vi "MesuresValiseCustomNeMarchePas.vi"() -> ()   [LabVIEW 2017]
uses:
  Globals/VarGlobUIStopLoops.vi
  <resource>/objmgr/daqmx.rc
  DefDeType/WhichPath.ctl
  <vilib>/DAQmx/write.llb/DAQmx Write (Digital Bool 1Line 1Point).vi
  <vilib>/DAQmx/create/channels.llb/DAQmx Create Channel (DO-Digital Output).vi
  DefDeType/ClusterRefCtrl.ctl
  <vilib>/DAQmx/read.llb/DAQmx Read (Analog 1D Wfm NChan NSamp).vi
panel:
  in  "Reprocess":bool
  in  "Next Test":u32
  out "AcqTime(s)":u16(slide) scale=0.0..1000.0
  out "Recording":bool
  in  "EnregistrerPtEtal":bool
  out "Projet":string
  in  "Essais réalisés":i32(listbox)
  out "Reload Config":bool
  out "Graph2":dbl[][](graph)
  in  "ChangerConfig":bool
  out "iterationMonitoringLoop":i32
  out "iterationEventLoop":i32
  in  "Stop Enreg.":bool
  in  "Enregistrer":bool
  out "Graph1":waveform(dbl)[](graph)
  in  "Quitter":bool
  # "Commandes"
  # "Graph 1"
  # "Essais Réalisés"
  # "Graph 2"
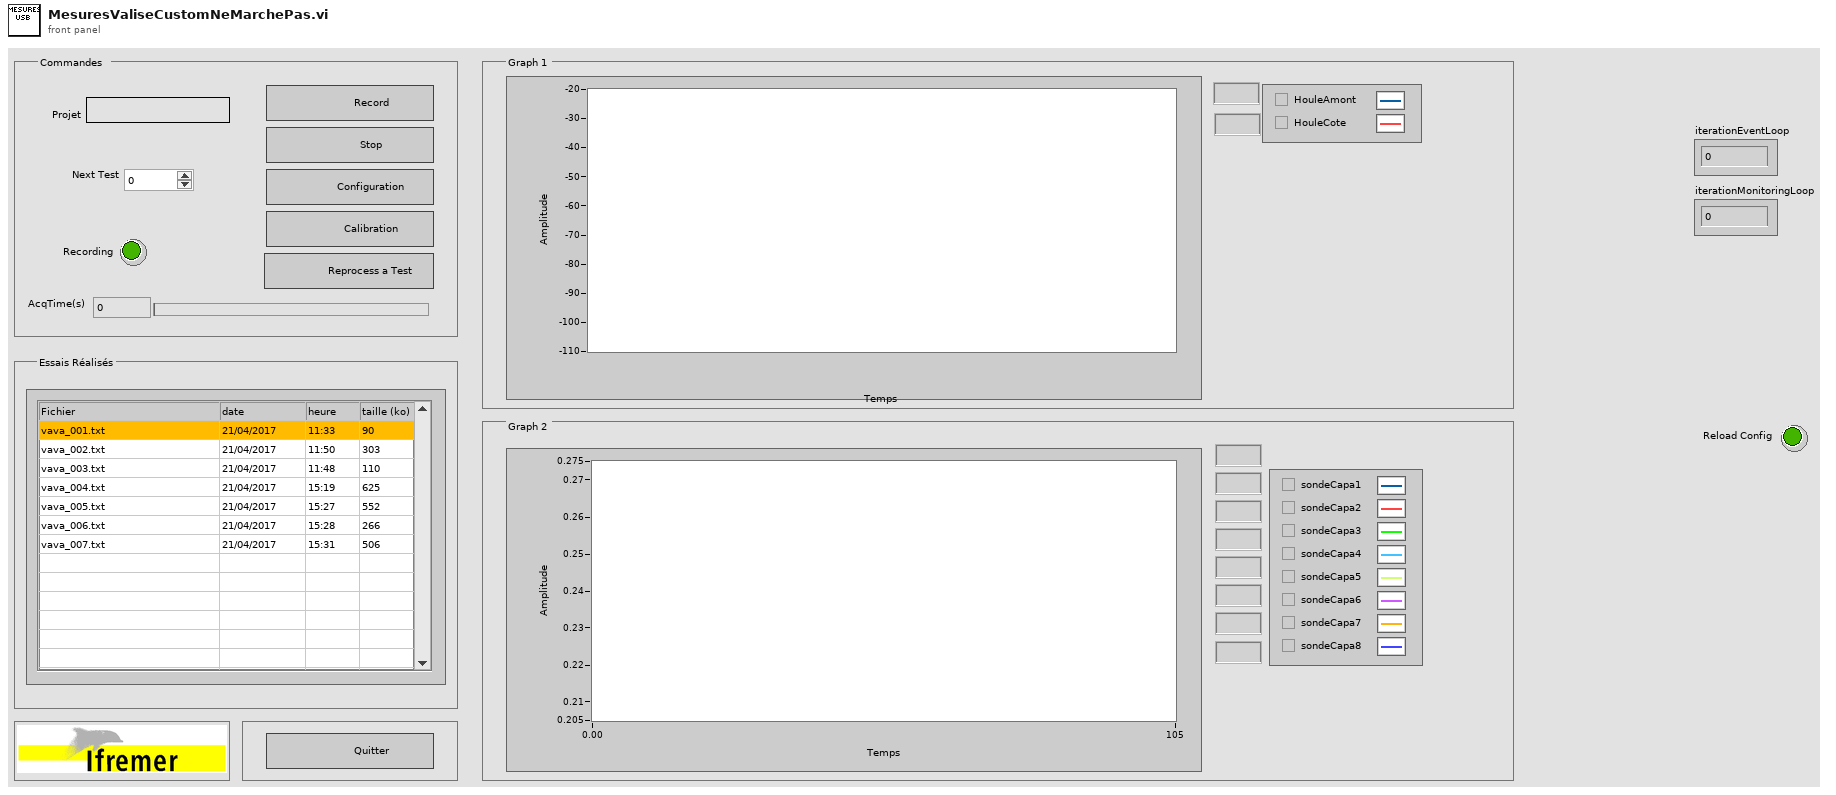
[diagram p1: front panel]
types:
  T1 = enum8{"Enabled", "Disabled", "Disabled and Grayed Out"}
  T2 = typedef "ClusterRefCtrl.ctl" = cluster{"Essais réalisés":refnum<vi>, "EnregistrerPtEtal":refnum<vi>, "ChangerConfig":refnum<vi>, "Enregistrer":refnum<vi>, "Reprocess":refnum<vi>}
  T3 = cluster{"AcqTime(s)":refnum<vi>, "Graph2":refnum<vi>, "Graph1":refnum<vi>}
  T4 = typedef "ConfigTotale.ctl" = cluster{"VoltageChannels":T5, "WheastoneBridgeChannels":T6, "Configuration":T7}
  T5 = typedef "VoltageChannels.ctl" = cluster{"ChannelNames":string[], "Sensitivity(Unit/V)":dbl[], "AutoZero":bool[], "ChannelUnits":string[], "Offsets(Units)":dbl[], "Graph Num":u8[]}
  T6 = typedef "WBridgeChannels.ctl" = cluster{"ChannelNames":string[], "Sensitivity(Unit/V)":dbl[], "AutoZero":bool[], "ChannelUnits":string[], "Offsets(Units)":dbl[], "Graph Num":u8[]}
  T7 = typedef "Configuration.ctl" = cluster{"AcqSamplingRate(Hz)":u32, "AcqTime(s)":u32, "Trigger":bool, "NbVoltageChannels":u32, "NbWBridgeChannels":u32, "Qualisys":bool, "Hexapode":bool, "FinalSamplingRate(Hz)":u32, "QualisysDataType":enum16{"6DOF", "3DTracking", "6DOF + 3D"}, "Nortek":bool, "HBM":bool}
  T8 = cluster{"Graph2Index":i32[], "Graph1Index":i32[]}
  T9 = typedef "WhichPath.ctl" = enum16{"DossierProjet", "Config", "Meas", "MeasPCI", "MeasCRIO1", "MeasCRIO2", "MeasQualisys", "MeasHBM", "MeasTDMS", "Fig", "Res"}
  T10 = typedef "MergeFileConfig.ctl" = cluster{"Test Num : ":u32, "Project :":string, "Qualisys file":path, "Hexapod file":path, "ADV Nortek file":path, "QualisysDataType":enum16{"6DOF", "3DTracking", "6DOF + 3D"}, "Qualisys":bool, "Hexapode":bool, "ADV Nortek":bool}
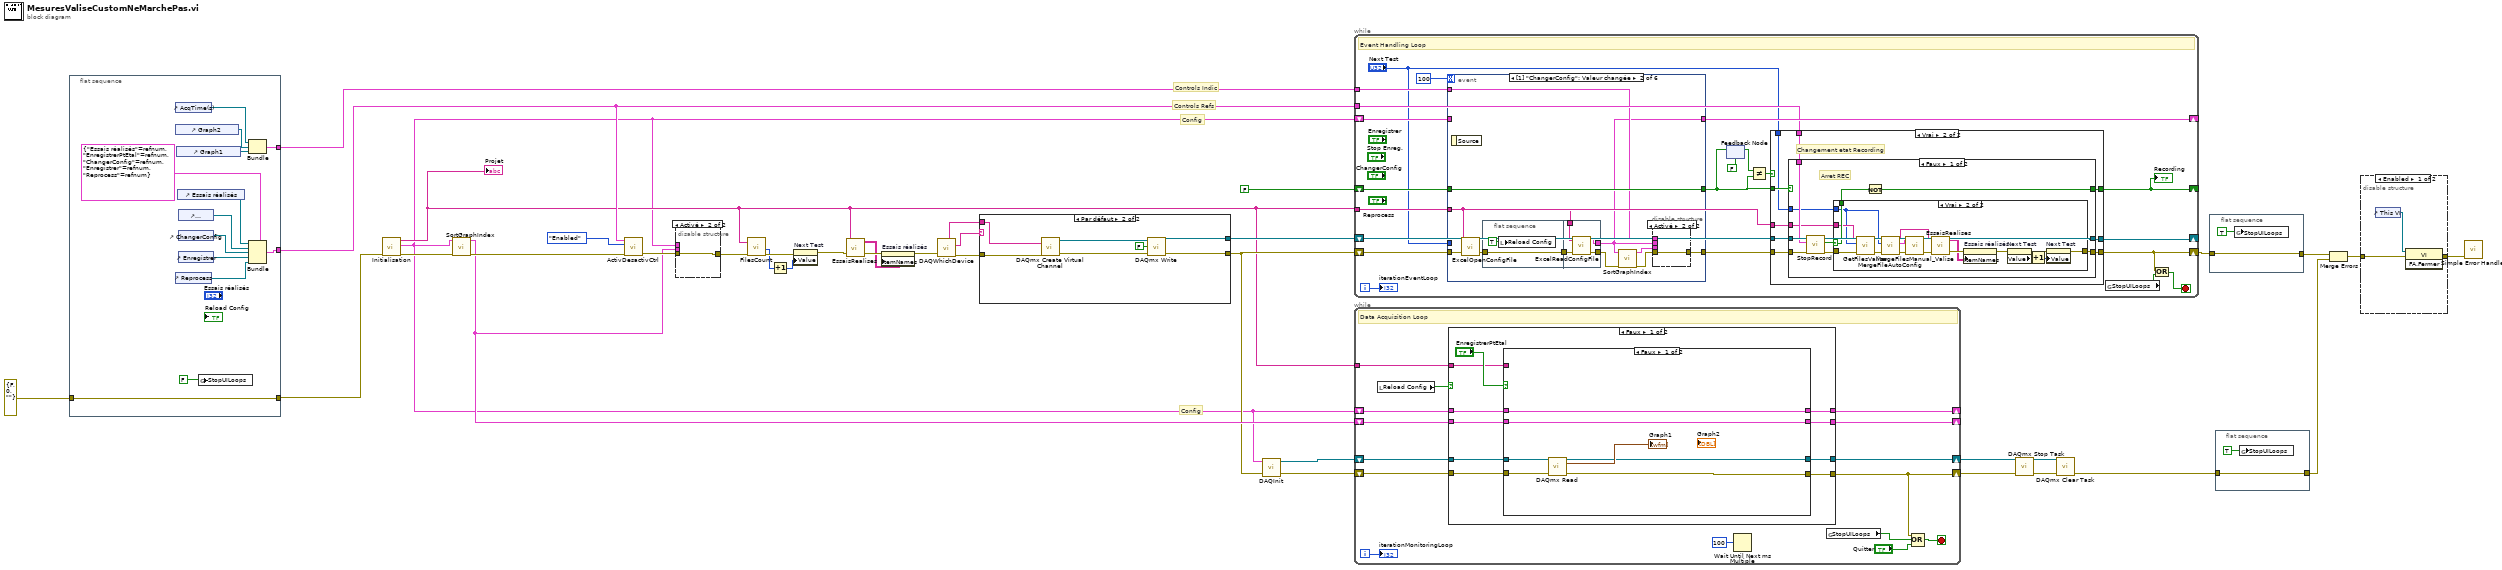
[diagram p0: block diagram]
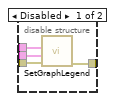
[diagram p2: hidden frame]
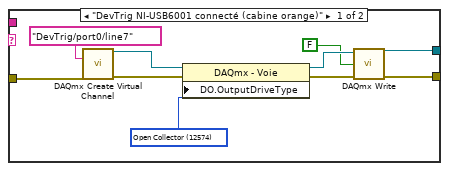
[diagram p4: hidden frame]
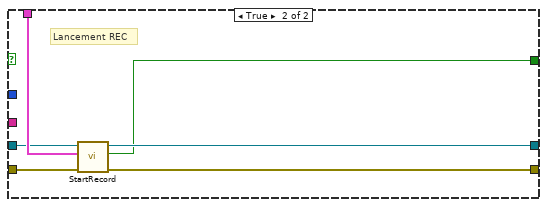
[diagram p7: hidden frame]
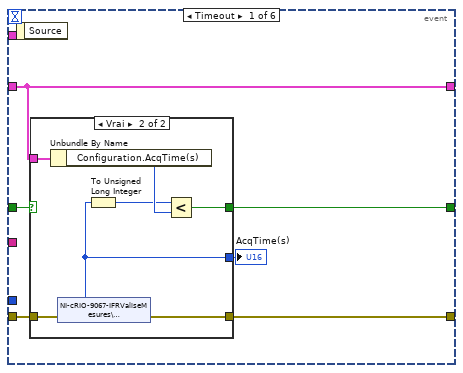
[diagram p8: hidden frame]
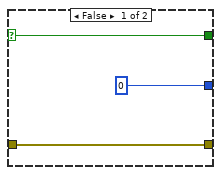
[diagram p9: hidden frame]
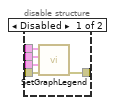
[diagram p10: hidden frame]
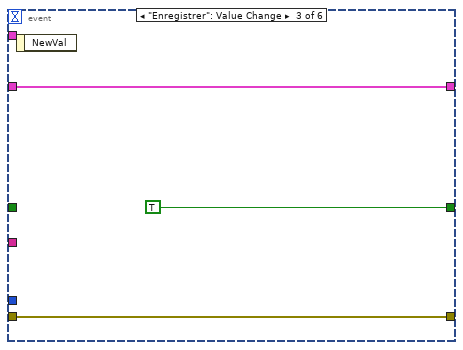
[diagram p11: hidden frame]
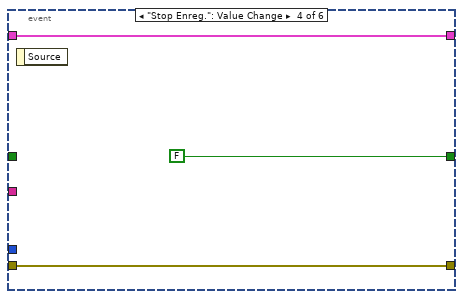
[diagram p12: hidden frame]
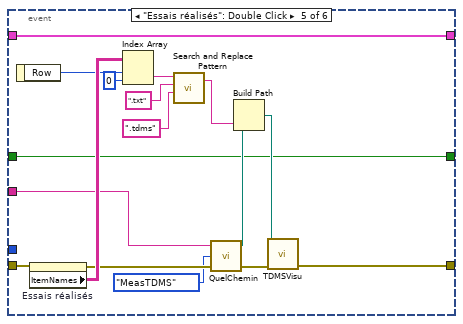
[diagram p13: hidden frame]
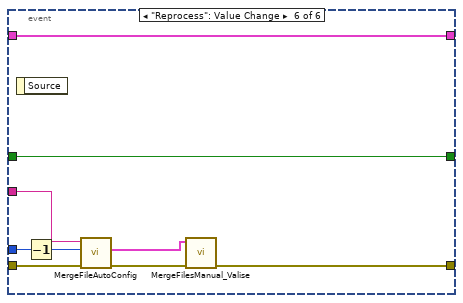
[diagram p14: hidden frame]
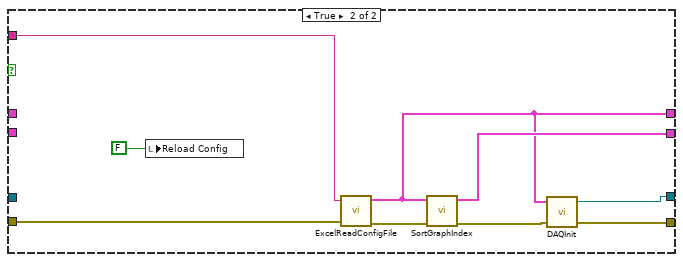
[diagram p16: hidden frame]
diagram:
  # "Controls Indic"
  # "Config"
  # "Config"
  # "Controls Refs"
  n1 = flat-sequence {
    tunnel: errorcluster {"status"=FALSE, "code"=0, "source"=""} ("entrée d'erreur (pas d'erreur)") -> [w38]
    tunnel: [w45] -> w30
    tunnel: [w41] -> w24
    tunnel: [w38] -> w16
    frame #0 {
      n2 = control-ref of="Graph2"() -> (w43:refnum<vi>)
      n3 = control-ref of="AcqTime(s)"() -> (w42:refnum<vi>)
      n4 = control-ref of="Reprocess"() -> (w39:refnum<vi>)
      n5 = control-ref of="Graph1"() -> (w44:refnum<vi>)
      n6 = control-ref of="Essais réalisés"() -> (w46:refnum<vi>)
      n7 = control-ref of="EnregistrerPtEtal"() -> (w47:refnum<vi>)
      n8 = control-ref of="ChangerConfig"() -> (w48:refnum<vi>)
      n9 = control-ref of="Enregistrer"() -> (w49:refnum<vi>)
      n10 = global write "VarGlobUIStopLoops.vi" "StopUILoops"(FALSE ("StopUILoops")) -> ()
      n11 = Bundle("AcqTime(s)"=w42, "Graph2"=w43, "Graph1"=w44) -> (w41:T3)  [unwired: 1 in]
      n12 = Bundle(cluster=T2 {"Essais réalisés"=refnum, "EnregistrerPtEtal"=refnum, "ChangerConfig"=refnum, "Enregistrer"=refnum, "Reprocess"=refnum} ("Cluster"), "Essais réalisés"=w46, "EnregistrerPtEtal"=w47, "ChangerConfig"=w48, "Enregistrer"=w49, "Reprocess"=w39) -> (w45:T2)
    }
  }
  n13 = call "Initialisation.vi"("Error In"=w16) -> ("Error Out"=w15:errorcluster, "ConfigurationTotale"=w1:T4, "NomProjetOUT"=w8:string)  [unwired: 4 in]
  "Projet" <- w8
  n14 = call "SortGraphIndex.vi"("Error In"=w15, "ConfigurationTotale"=w1) -> ("Error Out"=w14:errorcluster, "GraphIndex"=w13:T8)  [unwired: 4 in]
  n15 = call "ActivDesactivCtrl.vi"("error in (no error)"=w14, "Disabled"=T1."Enabled", "Cluster"=w30) -> ("error out"=w25:errorcluster)  [unwired: 4 in]
  n16 = disable-structure shown="Activé" {
    disable-tunnel: w25 -> [w54 w55]
    disable-tunnel: [w53 w55] -> w23
    disable-tunnel: w13 -> [w52 _]
    disable-tunnel: w1 -> [w51 _]
    frame Disabled {
      n17 = call "SetGraphLegend.vi"("error in (no error)"=w54, "GraphIndex"=w52, "ConfigTotale"=w51) -> ("error out"=w53:errorcluster)  [unwired: 4 in]
    }
    frame Enabled {
    }
  }
  n18 = call "FilesCount.vi"("NomProjet"=w8, "entrée d'erreur"=w23) -> ("NextTestNum"=w27:u32, "sortie d'erreur"=w29:errorcluster)  [unwired: 4 out]
  n19 = Increment(x=w27) -> (x+1=w26:u32)
  n20 = property on="Next Test" class="NumNb (strict)"(error in=w29, "Value"=w26) -> (error out=w28:errorcluster)  [unwired: 1 in, 1 out]
  n21 = call "EssaisRealises.vi"("entrée d'erreur (pas d'erreur)"=w28, "NomProjet"=w8) -> ("sortie d'erreur"=w33:errorcluster, "InfosFichiers"=w32:string[][])  [unwired: 2 in]
  n22 = property on="Essais réalisés" class="ListeMCol (strict)"(error in=w33, "ItemNames"=w32) -> (error out=w22:errorcluster)  [unwired: 1 in, 1 out]
  n23 = call "DAQWhichDevice.vi"("error in"=w22) -> ("error out"=w20:errorcluster, "Message"=w21:string, "DigitalInputFinAcq"=w19:tag)  [unwired: 1 in, 4 out]
  n24 = case shown="Par défaut" w21 {
    tunnel: [w59 w71] -> w10
    tunnel: [w58 w70] -> w31
    tunnel: w20 -> [w57 w69]
    tunnel: w19 -> [_ w66]
    frame "DevTrig NI-USB6001 connecté (cabine orange)" {
      w65 = 12574 items=["Active Drive"=12573, "Open Collector"=12574] ("DO.OutputDriveType")
      n25 = call-poly <vilib>:"DAQmx Create Virtual Channel.vi"("lines"=tag "DevTrig/port0/line7", "error in"=w57) -> ("task out"=w63:refnum<k21>, "error out"=w64:errorcluster)  [unwired: 12 in]
      n26 = property class="DAQmx - Voie"(reference=w63, error in=w64, "DO.OutputDriveType"=w65) -> (reference out=w61:refnum<k21>, error out=w60:errorcluster)
      n27 = call-poly <vilib>:"DAQmx Write.vi"("task/channels in"=w61, "data"=FALSE ("RecStarted"), "error in"=w60) -> ("task out"=w58:refnum<k21>, "error out"=w59:errorcluster)  [unwired: 10 in, 1 out]
    }
    frame Default {
      n28 = call-poly <vilib>:"DAQmx Create Virtual Channel.vi"("lines"=w66, "error in"=w69) -> ("task out"=w67:refnum<k21>, "error out"=w68:errorcluster)  [unwired: 12 in]
      n29 = call-poly <vilib>:"DAQmx Write.vi"("task/channels in"=w67, "data"=FALSE, "error in"=w68) -> ("task out"=w70:refnum<k21>, "error out"=w71:errorcluster)  [unwired: 10 in, 1 out]
    }
  }
  n30 = call "DAQInit.vi"("error in"=w10, "configInput"=w1) -> ("error out"=w9:errorcluster, "task out"=w7:refnum<k21>)  [unwired: 2 in]
  n31 = while {
    shift-right: [w81] -> w36
    shift-left: w10 -> [w92]
    tunnel: w8 -> [w75]
    shift-right: [w78] -> _
    shift-left: FALSE ("RecStarted") -> [w88]
    tunnel: w30 -> [w80]
    shift-right: [w86] -> _
    shift-left: w1 -> [w87]
    shift-right: [w82] -> _
    shift-left: w31 -> [w74]
    tunnel: w24 -> [w76]
    i -> [w91]
    stop <- w89 stop-if-true
    # "Event Handling Loop"
    n32 = event shown="[1] \"ChangerConfig\": Valeur changée" {
      selector: _ -> [_ _ _ _ _ _]
      dyn-events: _ -> [_ _ _ _ _ _]
      timeout: 100 -> [_ _ _ _ _ _]
      tunnel: w92 -> [w146 w168 w183 w186 w200 w209]
      tunnel: [w145 w162 w183 w186 w196 w210] -> w83
      tunnel: w75 -> [_ w166 _ _ w193 w208]
      tunnel: [w143 w167 TRUE ("recording?") FALSE ("recording?") w187 w211] -> w79
      tunnel: w88 -> [w147 w167 _ _ w187 w211]
      tunnel: w87 -> [w142 _ w181 w184 w188 w212]
      tunnel: [w142 w159 w181 w184 w188 w212] -> w86
      tunnel: w76 -> [_ w163 _ _ _ _]
      tunnel: "Next Test" -> [_ _ _ _ _ w207]
      event Timeout {
        n33 = event-data() -> ()  [unwired: 1 in, 1 out]
        n34 = case shown="Vrai" w147 {
          selector: w147 -> [w148 _]
          tunnel: w146 -> [w150 w157]
          tunnel: [w150 w156] -> w145
          tunnel: w142 -> [_ w155]
          tunnel: [u16 0 ("UInt16") w151] -> w144
          tunnel: [w148 w152] -> w143
          frame False {
          }
          frame True {
            n35 = Unbundle By Name(w155) -> ("Configuration.AcqTime(s)"=w154:u32)
            n36 = shared-variable "NI-cRIO-9067-IFRValiseMesures\\Bibliothèque2Variables.lvlib\\AcqTime"(error in=w157) -> (w151:u16, error out=w156:errorcluster)
            n37 = To Unsigned Long Integer(number=w151) -> (unsigned 32bit integer=w153:u32)
            n38 = Less?(x=w153, y=w154) -> (x < y?=w152:bool)
          }
        }
        "AcqTime(s)" <- w144
      }
      event "ChangerConfig": Value Change {
        n39 = event-data() -> ()  [unwired: 1 in, 1 out]
        n40 = call "ExcelOpenConfigFile.vi"("error in (no error)"=w168, "NomProjet"=w166) -> ("sortie d'erreur"=w164:errorcluster)  [unwired: 2 in, 1 out]
        n41 = flat-sequence {
          tunnel: w164 -> [w176]
          tunnel: [w176] -> w165
          tunnel: [w179] -> w158
          tunnel: w165 -> [w180]
          tunnel: w166 -> [w178]
          tunnel: [w177] -> w159
          frame #0 {
            n42 = local write "Reload Config"(TRUE ("Reload Config")) -> ()
          }
          frame #1 {
            n43 = call "ExcelReadConfigFile.vi"("NomProjet"=w178, "error in (no error)"=w180) -> ("ConfigurationTotale"=w177:T4, "error out"=w179:errorcluster)  [unwired: 3 in]
          }
        }
        n44 = call "SortGraphIndex.vi"("Error In"=w158, "ConfigurationTotale"=w159) -> ("Error Out"=w161:errorcluster, "GraphIndex"=w160:T8)  [unwired: 4 in]
        n45 = disable-structure shown="Activé" {
          disable-tunnel: w163 -> [w173 _]
          disable-tunnel: [w172 w174] -> w162
          disable-tunnel: w161 -> [w171 w174]
          disable-tunnel: w160 -> [w170 _]
          disable-tunnel: w159 -> [w169 _]
          frame Disabled {
            n46 = call "SetGraphLegend.vi"("error in (no error)"=w171, "GraphIndex"=w170, "ConfigTotale"=w169, "ClusterRefGraphs"=w173) -> ("error out"=w172:errorcluster)  [unwired: 3 in]
          }
          frame Enabled {
          }
        }
      }
      event "Enregistrer": Value Change {
        n47 = event-data() -> ()  [unwired: 1 in, 1 out]
      }
      event "Stop Enreg.": Value Change {
        n48 = event-data() -> ()  [unwired: 1 in, 1 out]
      }
      event "Essais réalisés": Double Click {
        n49 = event-data() -> ("Row"=w197:i32)  [unwired: 1 in]
        n50 = property on="Essais réalisés" class="ListeMCol (strict)"(error in=w200) -> (error out=w194:errorcluster, "ItemNames"=w199:string[][])  [unwired: 1 in, 1 out]
        n51 = Index Array(array=w199, index (row)=w197, index (col)=0 ("indice désactivé (col)")) -> (element=w201:string)
        n52 = call <vilib>:"Search and Replace Pattern.vi"("string"=w201, "regular expression (\"\")"=".txt" ("regular expression (\"\")"), "replace string (\"\")"=".tdms" ("replace string (\"\")")) -> ("result string"=w190:string)  [unwired: 2 in, 1 out]
        n53 = call "QuelChemin.vi"("Entrée d'erreur"=w194, "WhichPath?"=WhichPath."MeasTDMS", "NomProjet"=w193) -> ("Sortie d'erreur"=w195:errorcluster, "SurDisqueLocal"=w191:path)  [unwired: 1 out]
        n54 = Build Path(base path=w191, name or relative path=w190) -> (appended path=w189:path)
        n55 = call "TDMSVisu.vi"("error in (no error)"=w195, "file path"=w189) -> ("error out"=w196:errorcluster)  [unwired: 4 in, 1 out]
      }
      event "Reprocess": Value Change {
        n56 = event-data() -> ()  [unwired: 1 in, 1 out]
        n57 = Decrement(x=w207) -> (x-1=w204:u32)
        n58 = call "MergeFileAutoConfig.vi"("error in (no error)"=w209, "test num"=w204, "ProjetIN"=w208) -> ("error out"=w206:errorcluster, "MergeFileConfigOUT"=w205:T10)  [unwired: 2 in, 1 out]
        n59 = call "MergeFilesManual_Valise.vi"("Error In"=w206, "MergeFileConfINPUT"=w205) -> ("sortie d'erreur"=w210:errorcluster)  [unwired: 5 in]
      }
    }
    n60 = feedback-in #1(w79) -> ()
    n61 = feedback #1(FALSE ("recording?")) -> (w85:bool)
    n62 = Not Equal?(x=w85, y=w79) -> (x != y?=w84:bool)
    n63 = case shown="Vrai" w84 {
      tunnel: [w95 w100] -> w81
      tunnel: w83 -> [w95 w104]
      tunnel: [w96 w99] -> w82
      tunnel: w74 -> [w96 w105]
      tunnel: w80 -> [_ w103]
      tunnel: w79 -> [w94 w102]
      tunnel: [w94 w101] -> w78
      tunnel: "Next Test" -> [_ w98]
      tunnel: w75 -> [_ w97]
      frame False {
      }
      frame True {
        # "Changement etat Recording"
        n64 = case shown="Faux" w102 {
          tunnel: w105 -> [w115 w138]
          tunnel: w104 -> [w116 w141]
          tunnel: w103 -> [w114 w139]
          tunnel: [w112 w136] -> w101
          tunnel: [w109 w140] -> w100
          tunnel: [w113 w137] -> w99
          tunnel: w98 -> [w107 _]
          tunnel: w97 -> [w106 _]
          frame False {
            # "Arret REC"
            n65 = call "StopRecord.vi"("error in (no error)"=w116, "ClusterRefCtrlIN"=w114, "task/channels in"=w115) -> ("error out"=w110:errorcluster, "RecStopped"=w111:bool, "task out"=w113:refnum<k21>)  [unwired: 2 in]
            n66 = case shown="Vrai" w111 {
              selector: w111 -> [w117 w135]
              tunnel: w110 -> [w118 w126]
              tunnel: [w118 w130] -> w109
              tunnel: [w117 w135] -> w108
              tunnel: w107 -> [_ w123]
              tunnel: w106 -> [_ w127]
              frame False {
              }
              frame True {
                n67 = call "GetFilesValise.vi"("error in (no error)"=w126, "Test Num :"=w123, "Project :"=w127) -> ("error out"=w124:errorcluster, "NomProjetOut"=w125:string)  [unwired: 3 in]
                n68 = call "MergeFileAutoConfig.vi"("error in (no error)"=w124, "test num"=w123, "ProjetIN"=w125) -> ("error out"=w121:errorcluster, "MergeFileConfigOUT"=w119:T10, "ProjetOUT"=w122:string)  [unwired: 2 in]
                n69 = call "MergeFilesManual_Valise.vi"("Error In"=w121, "MergeFileConfINPUT"=w119) -> ("sortie d'erreur"=w120:errorcluster)  [unwired: 5 in]
                n70 = call "EssaisRealises.vi"("entrée d'erreur (pas d'erreur)"=w120, "NomProjet"=w122) -> ("sortie d'erreur"=w134:errorcluster, "InfosFichiers"=w133:string[][])  [unwired: 2 in]
                n71 = property on="Essais réalisés" class="ListeMCol (strict)"(error in=w134, "ItemNames"=w133) -> (error out=w132:errorcluster)  [unwired: 1 in, 1 out]
                n72 = property on="Next Test" class="NumNb (strict)"(error in=w132) -> (error out=w131:errorcluster, "Value"=w129:u32)  [unwired: 1 in, 1 out]
                n73 = Increment(x=w129) -> (x+1=w128:u32)
                n74 = property on="Next Test" class="NumNb (strict)"(error in=w131, "Value"=w128) -> (error out=w130:errorcluster)  [unwired: 1 in, 1 out]
              }
            }
            n75 = Not(x=w108) -> (.not. x?=w112:bool)
          }
          frame True {
            # "Lancement REC"
            n76 = call "StartRecord.vi"("error in (no error)"=w141, "ClusterRefCtrlIN"=w139, "task/channels in"=w138) -> ("error out"=w140:errorcluster, "RecStarted"=w136:bool, "task out"=w137:refnum<k21>)  [unwired: 2 in]
          }
        }
      }
    }
    "Recording" <- w78
    n77 = global read "VarGlobUIStopLoops.vi" "StopUILoops"() -> (w90:bool)
    n78 = Or(x=w81, y=w90) -> (x .or. y?=w89:bool)
    "iterationEventLoop" <- w91
  }
  n79 = while {
    shift-right: [w221] -> w6
    shift-left: w9 -> [w226]
    shift-right: [w218] -> _
    shift-left: w1 -> [w220]
    tunnel: w8 -> [w217]
    shift-right: [w216] -> _
    shift-left: w13 -> [w215]
    shift-right: [w213] -> w3
    shift-left: w7 -> [w214]
    i -> [w225]
    stop <- w224 stop-if-true
    # "Data Acquisition Loop"
    n80 = local read "Reload Config"() -> (w219:bool)
    n81 = case shown="Faux" w219 {
      tunnel: w226 -> [w237 w257]
      tunnel: [w236 w251] -> w221
      tunnel: w220 -> [w235 _]
      tunnel: [w234 w250] -> w218
      tunnel: w217 -> [w232 w256]
      tunnel: [w230 w253] -> w216
      tunnel: w215 -> [w231 _]
      tunnel: w214 -> [w229 _]
      tunnel: [w228 w249] -> w213
      frame False {
        n82 = case shown="Faux" "EnregistrerPtEtal" {
          tunnel: w237 -> [w242 w245]
          tunnel: [w239 w245] -> w236
          tunnel: w235 -> [w244 w248]
          tunnel: [w244 w248] -> w234
          tunnel: w232 -> [_ _]
          tunnel: w231 -> [w243 w247]
          tunnel: [w243 w247] -> w230
          tunnel: w229 -> [w240 w246]
          tunnel: [w238 w246] -> w228
          frame False {
            n83 = call-poly <vilib>:"DAQmx Read.vi"("task/channels in"=w240, "error in"=w242) -> ("task out"=w238:refnum<k21>, "data"=→"Graph1":waveform(dbl)[], "error out"=w239:errorcluster)  [unwired: 11 in]
          }
          frame True {
          }
        }
      }
      frame True {
        n84 = local write "Reload Config"(FALSE ("Reload Config")) -> ()
        n85 = call "ExcelReadConfigFile.vi"("NomProjet"=w256, "error in (no error)"=w257) -> ("ConfigurationTotale"=w250:T4, "error out"=w254:errorcluster)  [unwired: 3 in]
        n86 = call "SortGraphIndex.vi"("Error In"=w254, "ConfigurationTotale"=w250) -> ("Error Out"=w252:errorcluster, "GraphIndex"=w253:T8)  [unwired: 4 in]
        n87 = call "DAQInit.vi"("error in"=w252, "configInput"=w250) -> ("error out"=w251:errorcluster, "task out"=w249:refnum<k21>)  [unwired: 2 in]
      }
    }
    n88 = Wait Until Next ms Multiple(millisecond multiple=u32 100 ("n millisecondes")) -> ()  [unwired: 1 out]
    n89 = global read "VarGlobUIStopLoops.vi" "StopUILoops"() -> (w223:bool)
    n90 = Compound Arithmetic op=OR ("Opérateur arithmétique")(w221, w223, "Quitter") -> (w224:bool)
    "iterationMonitoringLoop" <- w225
  }
  n91 = call <vilib>:"DAQmx Stop Task.vi"("task/channels in"=w3, "error in"=w6) -> ("task out"=w2:refnum<k21>, "error out"=w5:errorcluster)  [unwired: 12 in]
  n92 = call <vilib>:"DAQmx Clear Task.vi"("task in"=w2, "error in"=w5) -> ("error out"=w4:errorcluster)  [unwired: 13 in]
  n93 = flat-sequence {
    tunnel: w36 -> [w258]
    tunnel: [w258] -> w35
    frame #0 {
      n94 = global write "VarGlobUIStopLoops.vi" "StopUILoops"(TRUE ("StopUILoops")) -> ()
    }
  }
  n95 = flat-sequence {
    tunnel: w4 -> [w260]
    tunnel: [w260] -> w34
    frame #0 {
      n96 = global write "VarGlobUIStopLoops.vi" "StopUILoops"(TRUE ("StopUILoops")) -> ()
    }
  }
  n97 = Merge Errors(w35, w34) -> (w17:errorcluster)
  n98 = disable-structure shown="Enabled" {
    disable-tunnel: [w263 w265] -> w18
    disable-tunnel: w17 -> [w262 w265]
    frame Enabled {
      n99 = control-ref of="This VI"() -> (w264:refnum<vi>)
      n100 = invoke class="VI" method="FA.Fermer"(reference=w264, error in=w262) -> (error out=w263:errorcluster)  [unwired: 1 in, 2 out]
    }
    frame Disabled {
    }
  }
  n101 = call <vilib>:"Simple Error Handler.vi"("error in (no error)"=w18) -> ()  [unwired: 4 in, 5 out]
